vi "Read Version Number.vi"(8 "error in (no error)":errorcluster, 11 "Package Details in":refnum<class "Package Version.lvclass">) -> (0 "error out":errorcluster, 2 "Version Number":T1, 3 "Package Details out":refnum<class "Package Version.lvclass">)   [LabVIEW 2016, in "Packages.lvlib" / "Package Version.lvclass"]
uses:
  Package Version.lvclass
  Version Number--cluster.ctl
  Package Version.lvclass/Package Version.ctl
  Packages.lvlib
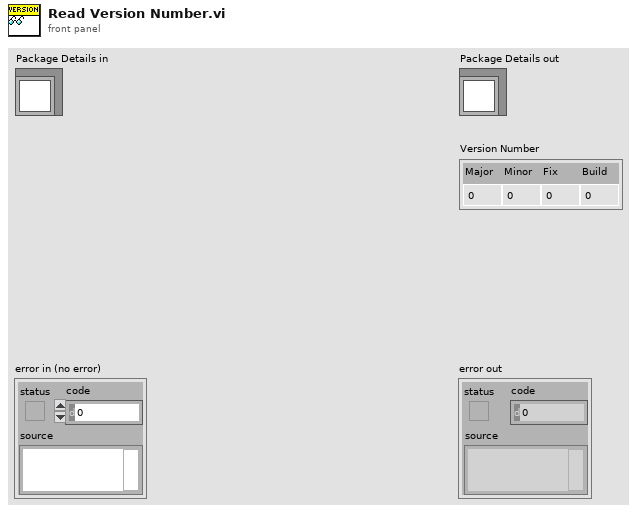
[diagram p1: front panel]
types:
  T1 = typedef "Packages.lvlib/Version Number--cluster.ctl" = cluster{"Major":i32, "Minor":i32, "Fix":i32, "Build":i32}
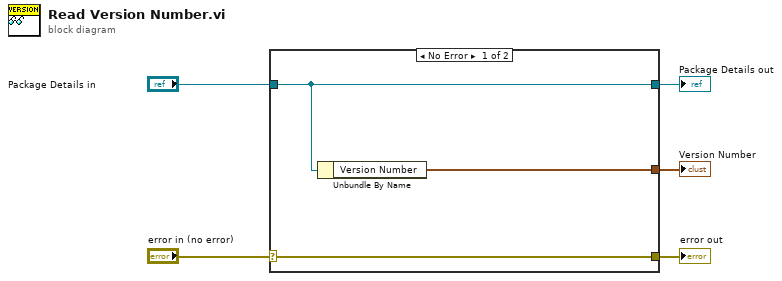
[diagram p0: block diagram]
diagram:
  n1 = case shown="No Error" "error in (no error)" {
    selector: "error in (no error)" -> [w8 w9]
    tunnel: [w8 w9] -> w4
    tunnel: [w7 w10] -> w2
    tunnel: "Package Details in" -> [w7 w10]
    tunnel: [w6 _] -> w1
    frame No Error {
      n2 = Unbundle By Name(w7) -> ("Version Number"=w6:T1)
    }
    frame Error {
    }
  }
  "error out" <- w4
  "Package Details out" <- w2
  "Version Number" <- w1
